vi "CRYView Pic Command Add.vi"(10 "cCommand":T1) -> ()   [LabVIEW 2013]
uses:
  CRYView Global.vi
panel:
  out "bResult":bool=TRUE
  out "Start_Positin 2":T2
  in  "ToolBar Click":bool
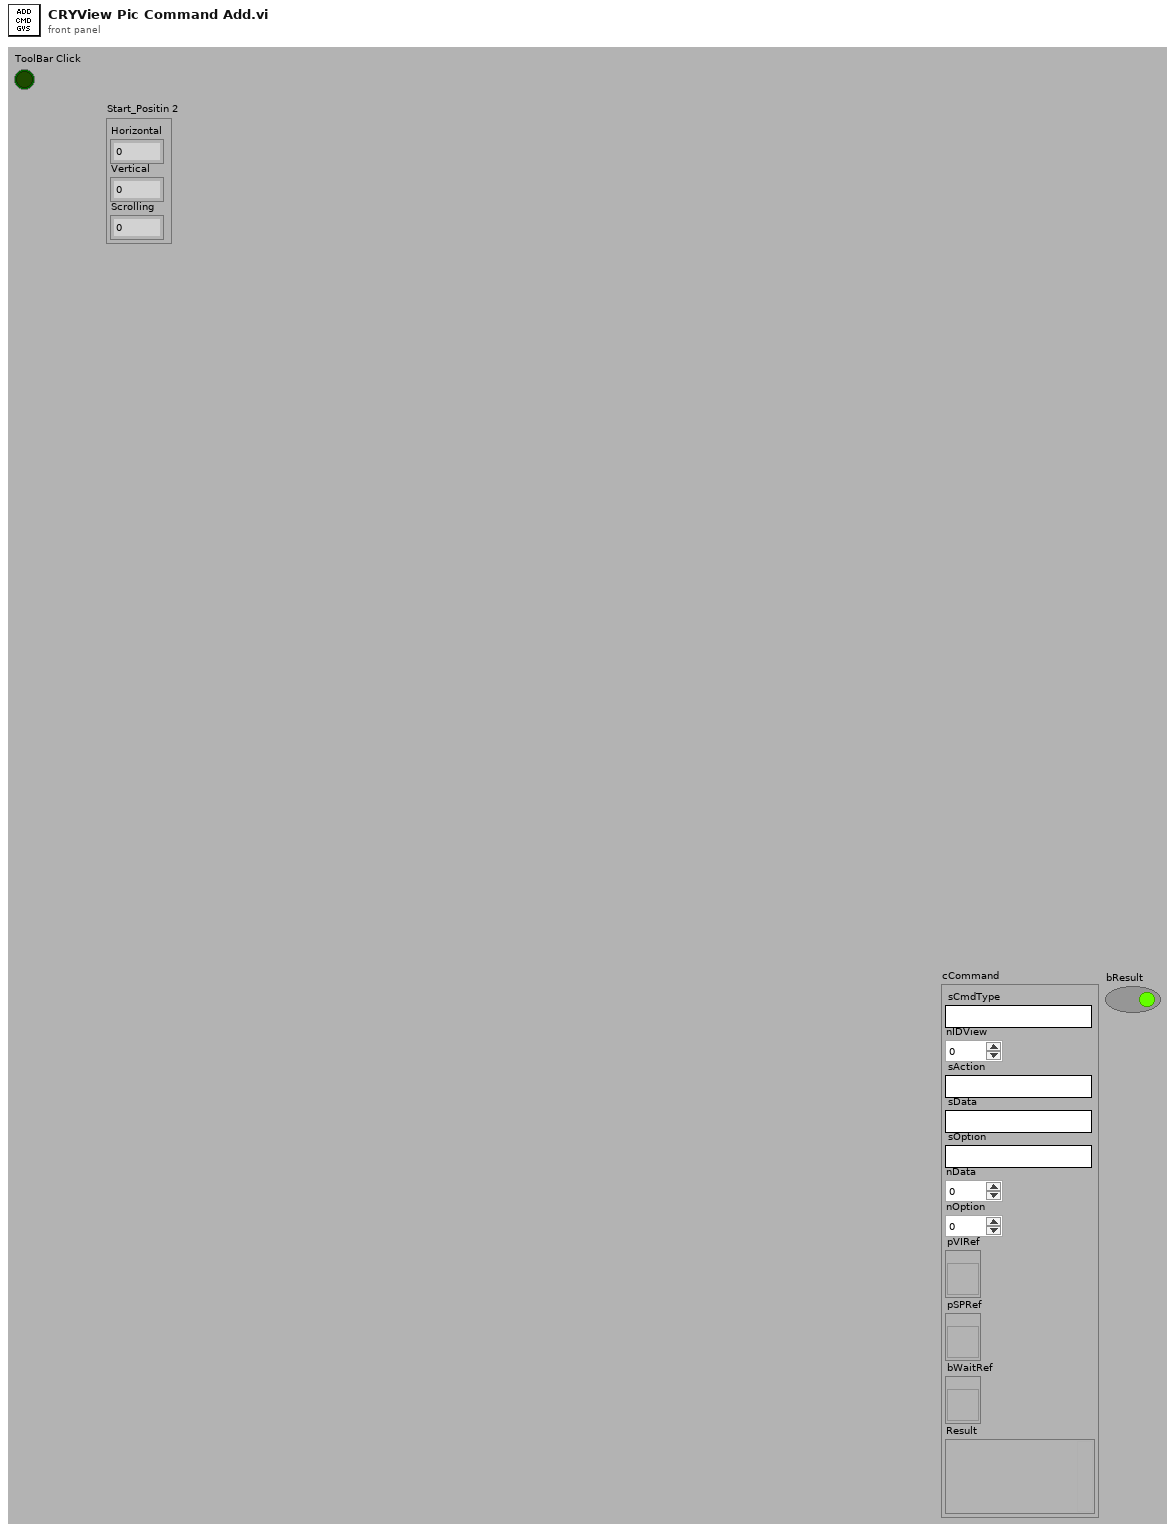
[diagram p1: front panel]
types:
  T1 = cluster{"sCmdType":string, "nIDView":i32, "sAction":string, "sData":string, "sOption":string, "nData":i32, "nOption":i32, "pVIRef":refnum<vi>, "pSPRef":refnum<vi>, "bWaitRef":refnum<vi>, "Result":variant}
  T2 = cluster{"Horizontal":i32, "Vertical":i32, "Scrolling":i32}
  T3 = cluster{"sCmdType":string, "nIDView":i32, "sAction":string, "sData":string, "sOption":string, "nData":i32, "nOption":i32, "pVIRef":refnum<vi>, "pSPRef":refnum<vi>, "bWaitRef":refnum<vi>, "Result":variant}[]
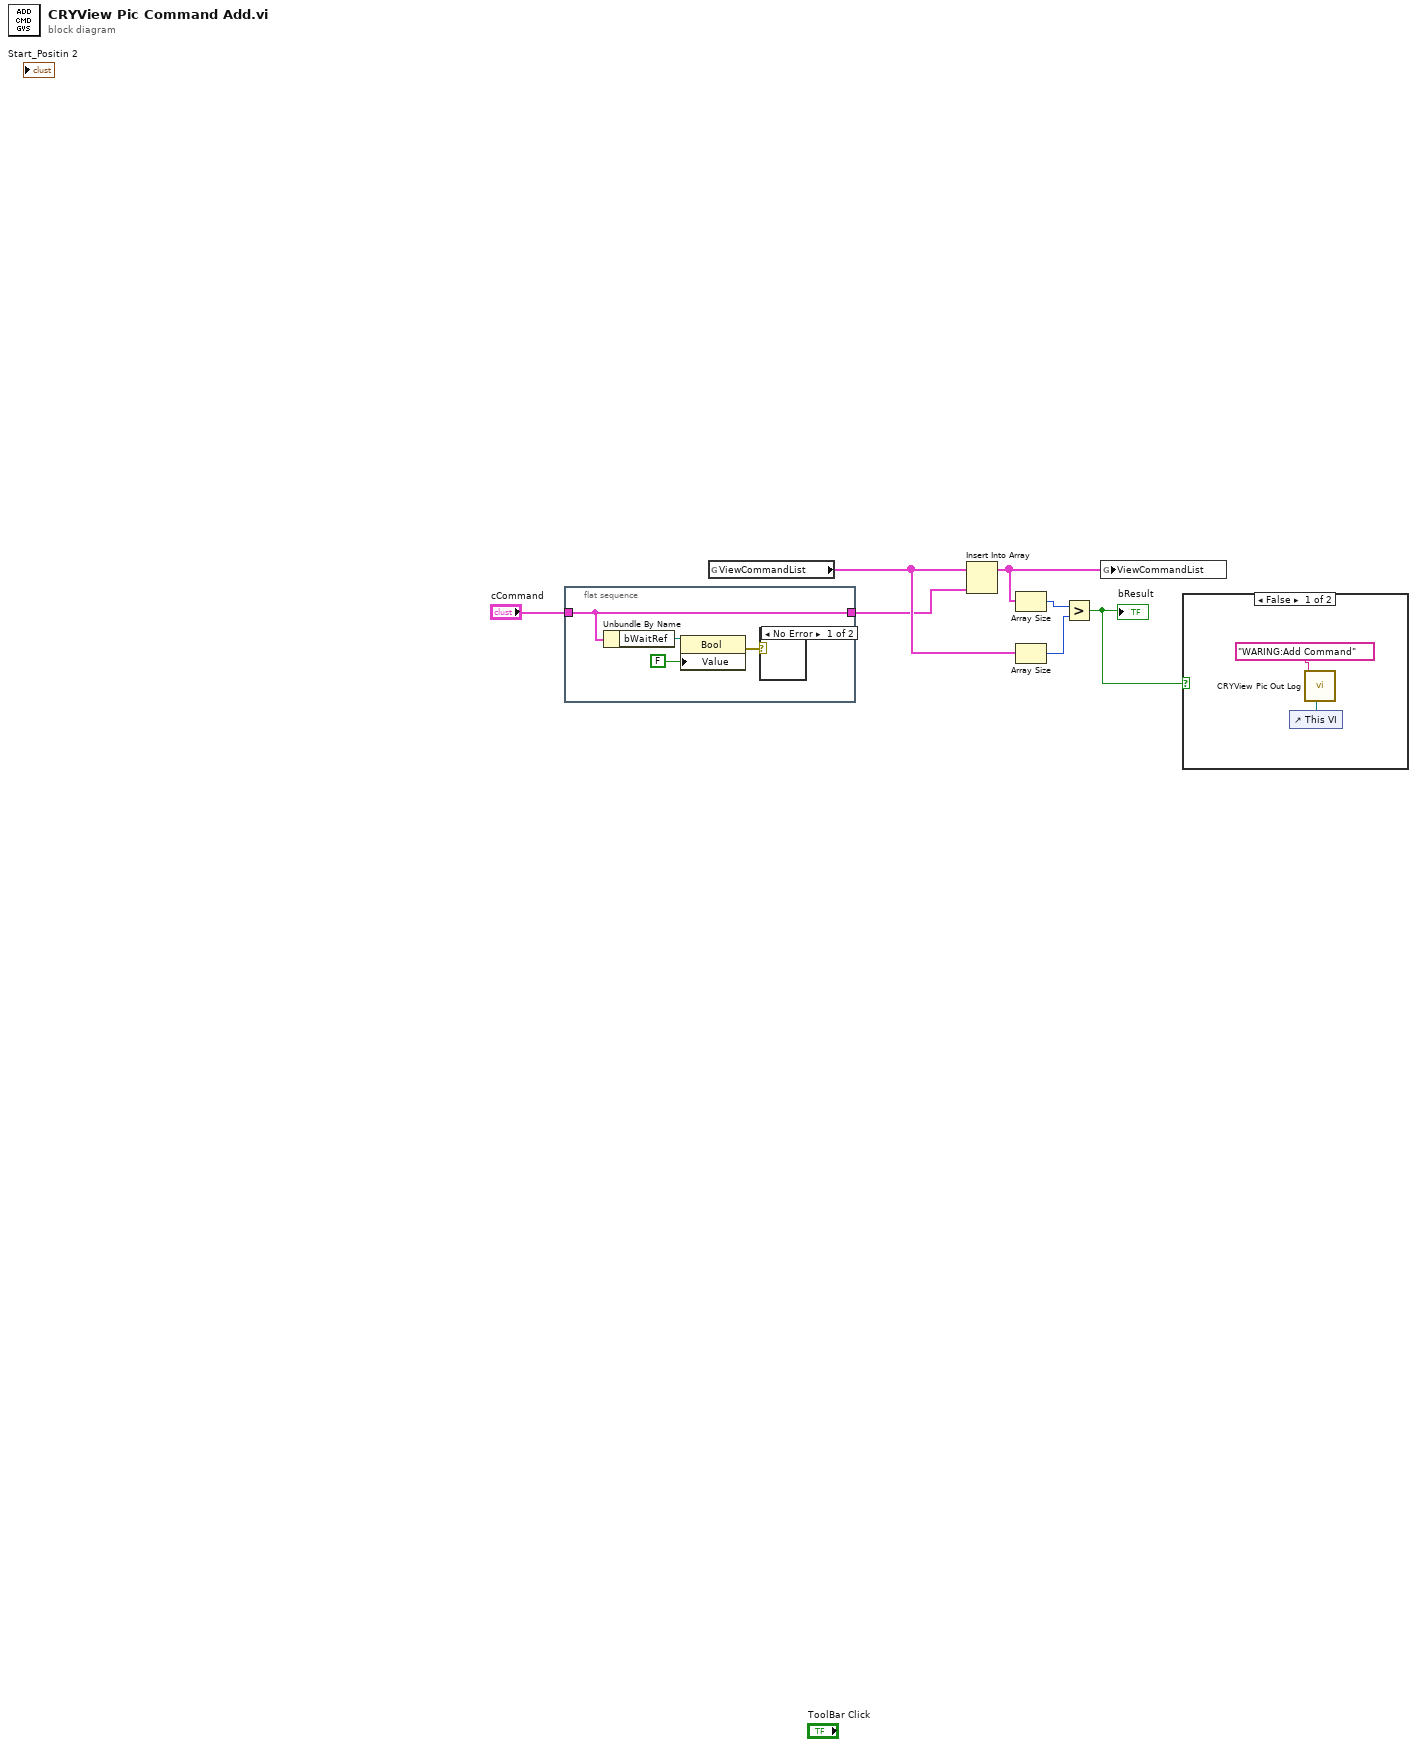
[diagram p0: block diagram]
diagram:
  n1 = flat-sequence {
    tunnel: "cCommand" -> [w9]
    tunnel: [w9] -> w1
    frame #0 {
      n2 = Unbundle By Name(w9) -> ("bWaitRef"=w11:refnum<vi>)
      n3 = property class="Bool"(reference=w11, "Value"=FALSE) -> (error out=w8:errorcluster)  [unwired: 1 in, 1 out]
      n4 = case shown="No Error" w8 {
        frame No Error {
        }
        frame Error {
        }
      }
    }
  }
  n5 = global read "CRYView Global.vi" "ViewCommandList"() -> (w7:T3)
  n6 = Insert Into Array(array=w7, new element=w1) -> (w4:T3)  [unwired: 1 in]
  n7 = Array Size(array=w4) -> (size(s)=w6:i32)
  n8 = Array Size(array=w7) -> (size(s)=w5:i32)
  n9 = Greater?(x=w6, y=w5) -> (0:w3:bool)
  "bResult" <- w3
  n10 = global write "CRYView Global.vi" "ViewCommandList"(w4) -> ()
  n11 = case shown="False" w3 {
    frame False {
      n12 = control-ref of="This VI"() -> (w13:refnum<vi>)
      n13 = call "CRYView Pic Out Log.vi"("vi reference"=w13, "sData"="WARING:Add Command") -> ()  [unwired: 10 in]
    }
    frame True {
    }
  }
